vi "Replace Line.vi"(8 "error in":errorcluster, 9 "New Line":T1 {"OPC UA Data Type" items=["Boolean"=1, "SByte"=2, "Byte"=3, "Int16"=4, "UInt16"=5, "Int32"=6, "UInt32"=7, "Int64"=8, "UInt64"=9, "Float"=10, "Double"=11, "String"=12, "DateTime"=13, "ByteString"=15, "Array of Boolean"=101, "Array of SByte"=102, "Array of Byte"=103, "Array of Int16"=104, "Array of UInt16"=105, "Array of Int32"=106, "Array of UInt32"=107, "Array of Int64"=108, "Array of UInt64"=109, "Array of Float"=110, "Array of Double"=111, "Array of String"=112, "Array of DateTime"=113, "Array of ByteString"=115]}, 10 "Line Name":string, 11 "OPC UA configuration in":refnum<class "OPC UA Client configuration.lvclass">) -> (0 "error out":errorcluster, 2 "Old Line":T1 {"OPC UA Data Type" items=["Boolean"=1, "SByte"=2, "Byte"=3, "Int16"=4, "UInt16"=5, "Int32"=6, "UInt32"=7, "Int64"=8, "UInt64"=9, "Float"=10, "Double"=11, "String"=12, "DateTime"=13, "ByteString"=15, "Array of Boolean"=101, "Array of SByte"=102, "Array of Byte"=103, "Array of Int16"=104, "Array of UInt16"=105, "Array of Int32"=106, "Array of UInt32"=107, "Array of Int64"=108, "Array of UInt64"=109, "Array of Float"=110, "Array of Double"=111, "Array of String"=112, "Array of DateTime"=113, "Array of ByteString"=115]}, 3 "OPC UA configuration out":refnum<class "OPC UA Client configuration.lvclass">)   [LabVIEW 2014, in "OPC UA Client configuration.lvclass"]
uses:
  OPC UA Client configuration.lvclass
  Line.ctl
  <vilib>/NI/Tag Bus Module Framework/channel/TBM channel.lvclass
  OPC UA Data Type.ctl
  OPC UA Client configuration.lvclass/OPC UA Client configuration.ctl
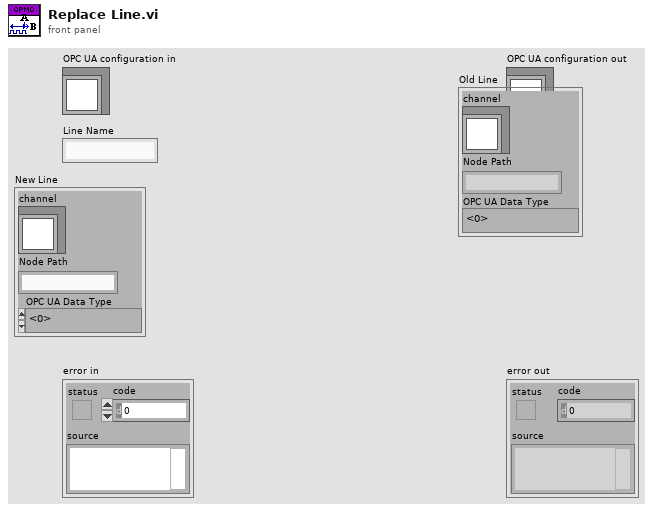
[diagram p1: front panel]
types:
  T1 = typedef "OPC UA Client configuration.lvclass/Line.ctl" = cluster{"channel":refnum<class "TBM channel.lvclass">, "Node Path":string, "OPC UA Data Type":T2}
  T2 = typedef "OPC UA Client configuration.lvclass/OPC UA Data Type.ctl" = u16
  T3 = cluster{"channel":refnum<class "TBM channel.lvclass">, "Node Path":string, "OPC UA Data Type":T2}[]
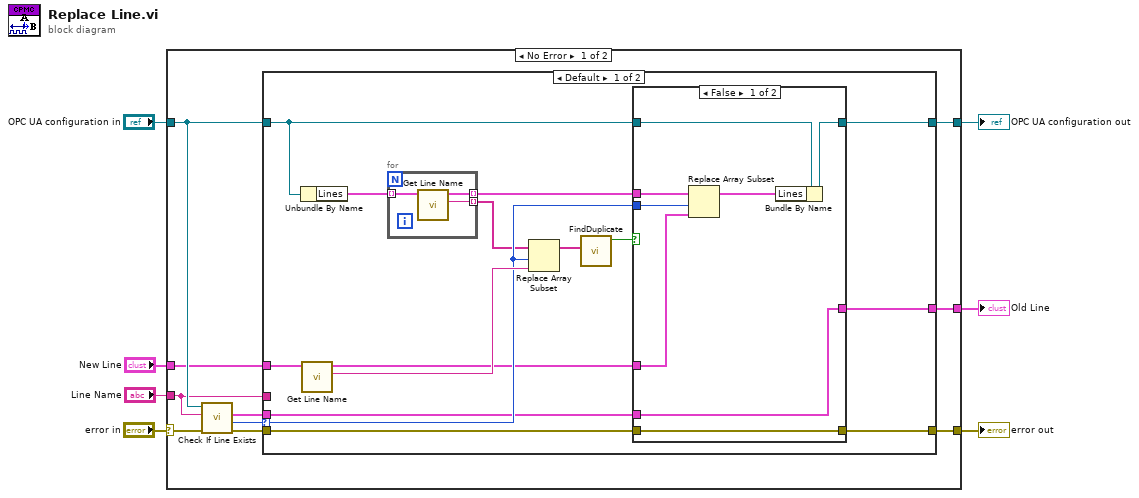
[diagram p0: block diagram]
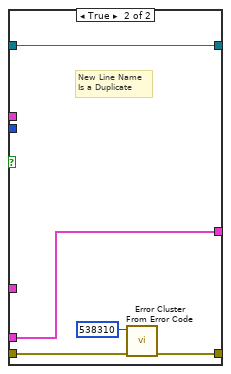
[diagram p2: hidden frame]
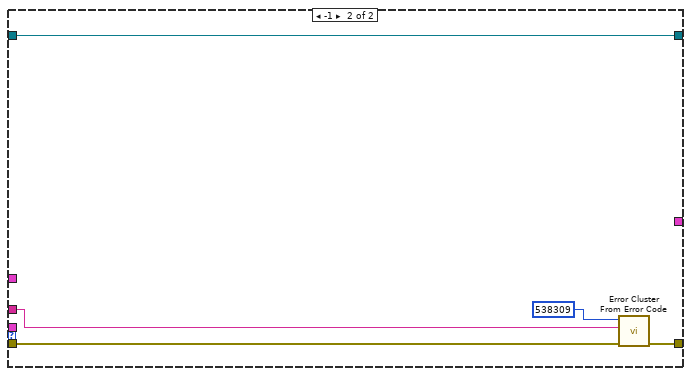
[diagram p3: hidden frame]
diagram:
  n1 = case shown="No Error" "error in" {
    selector: "error in" -> [w10 w55]
    tunnel: [w16 w55] -> w6
    tunnel: [w17 w54] -> w4
    tunnel: "OPC UA configuration in" -> [w15 w54]
    tunnel: "Line Name" -> [w14 _]
    tunnel: "New Line" -> [w12 _]
    tunnel: [w11 _] -> w1
    frame No Error {
      n2 = call-dynamic "Check If Line Exists.vi"("error in"=w10, "name to locate"=w14, "OPC UA configuration in"=w15) -> ("error out"=w9:errorcluster, "index"=w13:i32, "Line out"=w8:T1)  [unwired: 4 in, 2 out]
      n3 = case shown="Default" w13 {
        selector: w13 -> [w27 _]
        tunnel: w15 -> [w23 w53]
        tunnel: [w22 w53] -> w17
        tunnel: w12 -> [w31 _]
        tunnel: w14 -> [_ w51]
        tunnel: w9 -> [w25 w50]
        tunnel: [w24 w49] -> w16
        tunnel: [w20 _] -> w11
        tunnel: w8 -> [w21 _]
        frame Default {
          n4 = Unbundle By Name(w23) -> ("Lines"=w32:T3)
          n5 = call "Get Line Name.vi"("Line in"=w31) -> ("Name"=w30:string, "Line out"=w19:T1)  [unwired: 8 in, 1 out]
          n6 = for {
            tunnel: w32 -> [w48] mode=indexing
            tunnel: [w47] -> w18 mode=indexing
            tunnel: [w46] -> w26 mode=indexing
            n7 = call "Get Line Name.vi"("Line in"=w48) -> ("Name"=w46:string, "Line out"=w47:T1)  [unwired: 8 in, 1 out]
          }
          n8 = Replace Array Subset(array=w26, new element=w30, index=w27) -> (w29:string[])
          n9 = call "FindDuplicate.vi"("Array"=w29) -> ("Duplicate"=w28:bool)  [unwired: 8 in, 2 out]
          n10 = case shown="False" w28 {
            tunnel: w27 -> [w37 _]
            tunnel: w18 -> [w38 _]
            tunnel: w25 -> [w35 w45]
            tunnel: [w35 w44] -> w24
            tunnel: w23 -> [w40 w42]
            tunnel: [w39 w42] -> w22
            tunnel: w21 -> [w33 w41]
            tunnel: [w33 w41] -> w20
            tunnel: w19 -> [w34 _]
            frame False {
              n11 = Replace Array Subset(array=w38, new element=w34, index=w37) -> (w36:T1[])
              n12 = Bundle By Name(cluster=w40, "Lines"=w36) -> (w39:refnum<class "OPC UA Client configuration.lvclass">)
            }
            frame True {
              # "New Line Name\nIs a Duplicate"
              n13 = call <vilib>:"Error Cluster From Error Code.vi"("error in (no error)"=w45, "error code (0)"=538310) -> ("error out"=w44:errorcluster)  [unwired: 7 in]
            }
          }
        }
        frame -1 {
          n14 = call <vilib>:"Error Cluster From Error Code.vi"("error in (no error)"=w50, "error message (\"\")"=w51, "error code (0)"=538309) -> ("error out"=w49:errorcluster)  [unwired: 6 in]
        }
      }
    }
    frame Error {
    }
  }
  "error out" <- w6
  "OPC UA configuration out" <- w4
  "Old Line" <- w1
